vi "Create Data Channel - Array - Comparison.vi"(8 "error in (no error)":errorcluster, 9 "settings":T2, 10 "channel name":string, 11 "response refnum in":T1 format="%.0x") -> (0 "error out":errorcluster, 1 "channel refnums":T1[](array[typedef]) format="%.0x", 2 "array refnum":T1=18446744073709551615 format="%.0x", 3 "response refnum out":T1 format="%.0x")   [LabVIEW 2018, in "Instrument Addon Scripting API.lvlib"]
doc: "Creates a new Data Channel Array under the specified response."
uses:
  Instrument Addon Scripting API.lvlib
  Addon/Addon Shared/Types/Endian.ctl
  Addon/Addon Shared/Instrument Addon Shared.lvlib
  Addon/Addon Shared/Types/Type Cast Type.ctl
  Addon/Addon Shared/Types/Data Channel Type.ctl
  Addon/Addon Shared/Types/Protocol Data Type.ctl
  Addon/Addon Shared/Types/Data Parameters.ctl
  Addon/Addon Shared/SubVIs/Constants.vi
  <vilib>/NI Veristand/Custom Device API/Custom Device Item Ref.ctl
  <vilib>/NI Veristand/Custom Device API/Custom Device API.lvlib
  TypeDefs/Array Element.ctl
  TypeDefs/Array Comparison Settings.ctl
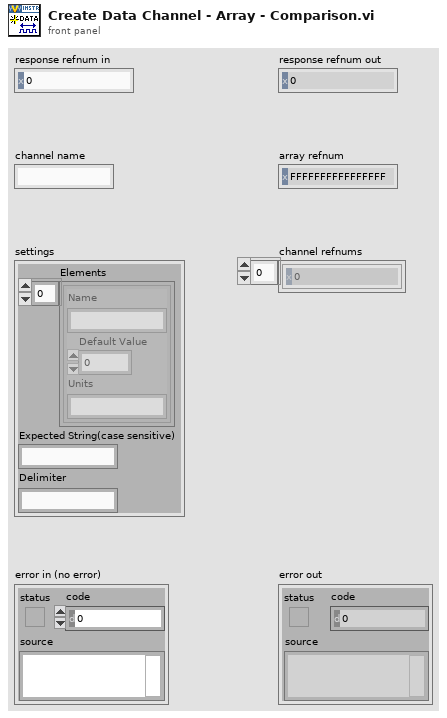
[diagram p1: front panel]
types:
  T1 = typedef "Custom Device API.lvlib/Custom Device Item Ref.ctl" = u64
  T2 = typedef "Instrument Addon Scripting API.lvlib/Array Comparison Settings.ctl" = cluster{"Elements":T3[], "Expected String(case sensitive)":string, "Delimiter":string}
  T3 = typedef "Instrument Addon Scripting API.lvlib/Array Element.ctl" = cluster{"Name":string, "Default Value":dbl, "Units":string}
  T4 = typedef "Instrument Addon Shared.lvlib/Data Channel Type.ctl" = enum16{"Format", "Comparison", "Type Cast", "Enumerated List"}
  T5 = typedef "Instrument Addon Shared.lvlib/Protocol Data Type.ctl" = enum16{"Single Channel", "Array"}
  T6 = typedef "Instrument Addon Shared.lvlib/Data Parameters.ctl" = cluster{"Data Type":T5, "Channel Type":T4, "Format String":string, "Expected String":string, "Type":T7, "List":string[], "Delimiter":string, "Endian":T8}
  T7 = typedef "Instrument Addon Shared.lvlib/Type Cast Type.ctl" = enum16{"DBL", "SGL", "U64", "U32", "U16", "U8", "I64", "I32", "I16", "I8"}
  T8 = typedef "Instrument Addon Shared.lvlib/Endian.ctl" = enum16{"Native", "Little", "Big"}
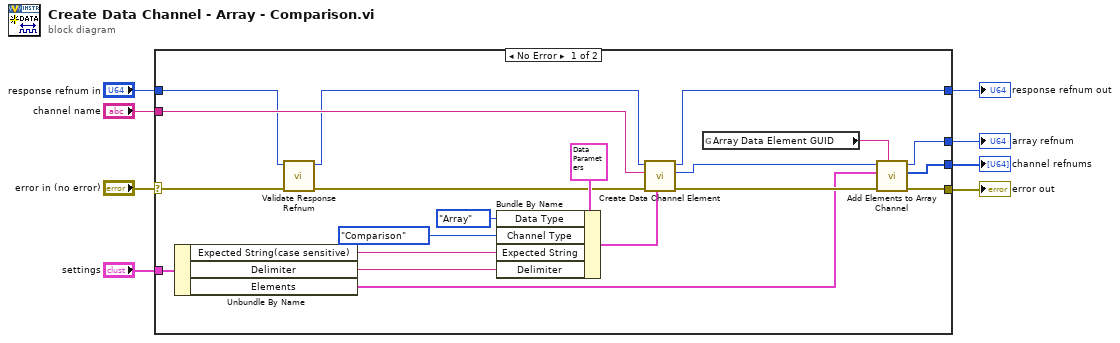
[diagram p0: block diagram]
diagram:
  n1 = case shown="No Error" "error in (no error)" {
    selector: "error in (no error)" -> [w13 w30]
    tunnel: [w24 w30] -> w8
    tunnel: [w15 w29] -> w7
    tunnel: "channel name" -> [w22 _]
    tunnel: "response refnum in" -> [w11 w29]
    tunnel: "settings" -> [w23 _]
    tunnel: [w16 _] -> w2
    tunnel: [w14 _] -> w1
    frame No Error {
      n2 = Unbundle By Name(w23) -> ("Expected String(case sensitive)"=w25:string, "Delimiter"=w17:string, "Elements"=w18:T3[])
      n3 = call "Validate Response Refnum.vi"("error in (no error)"=w13, "response refnum in"=w11) -> ("error out"=w12:errorcluster, "response refnum out"=w10:T1)  [unwired: 8 in]
      n4 = Bundle By Name(cluster=T6 {"Data Type"=enum."Array", "Channel Type"=enum."Format", "Format String"="%.3g", "Expected String"="", "Type"=enum."SGL", "List"=[], "Delimiter"=",", "Endian"=enum."Native"} ("Settings"), "Data Type"=Protocol_Data_Type."Array", "Channel Type"=Data_Channel_Type."Comparison", "Expected String"=w25, "Delimiter"=w17) -> (w21:T6)
      n5 = call "Create Data Channel Element.vi"("Data Channel Parameters"=w21, "Error In"=w12, "Name"=w22, "Refnum In"=w10) -> ("Error Out"=w20:errorcluster, "Channel Refnum"=w19:T1, "Refnum Out"=w15:T1)  [unwired: 5 in]
      n6 = global read "Constants.vi" "Array Data Element GUID"() -> (w9:string)
      n7 = call "Add Elements to Array Channel.vi"("array element GUID"=w9, "error in (no error)"=w20, "array elements"=w18, "array refnum in"=w19) -> ("error out"=w24:errorcluster, "channel refnums"=w16:T1[], "array refnum out"=w14:T1)  [unwired: 5 in]
    }
    frame Error {
    }
  }
  "error out" <- w8
  "response refnum out" <- w7
  "channel refnums" <- w2
  "array refnum" <- w1
